vi "LVObject to JSON.vi"(5 "enable LabVIEW extensions? (T)":bool=TRUE, 6 "Pretty Print?":bool, 7 "JSON Serializable Serializer in":refnum<class "JSON Serializable Serializer.lvclass">, 8 "error in (no error)":errorcluster, 10 "Object":refnum<class>) -> (0 "error out":errorcluster, 2 "<JSON>Object":string)   [LabVIEW 2017, in "JSON Serializable Serializer.lvclass"]
uses:
  JSON Serializable Serializer.lvclass
  C:/Program Files (x86)/National Instruments/LabVIEW 2017/vi.lib/JDP Science/JSONtext/LVClass Serializer/JSONtext LVClass Serializer.lvclass
  JSON Serializable/JSON Serializable.lvclass
  Default Serialization Binder/Default Serialization Binder.lvclass
  <vilib>/JDP Science/JSONtext/Set Multiple Object Items.vi
  <vilib>/JDP Science/JSONtext/Get all Object Items.vi
  <vilib>/JDP Science/JSONtext/JSON type.vi
  <vilib>/JDP Science/JSONtext/JSONtext.lvlib
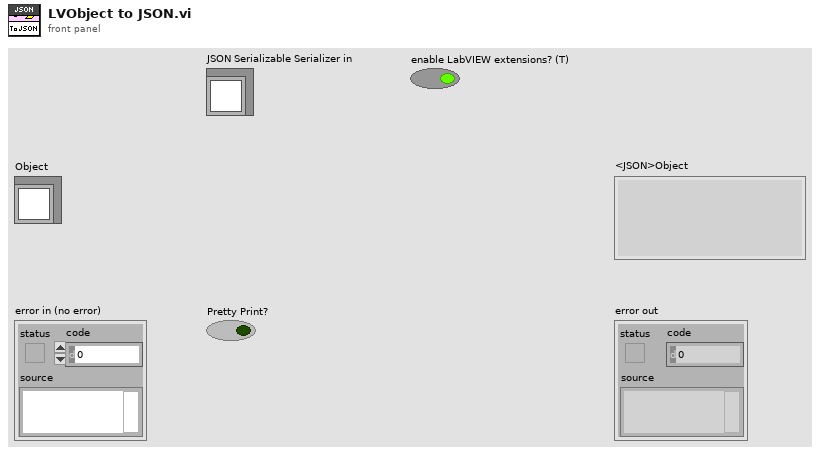
[diagram p1: front panel]
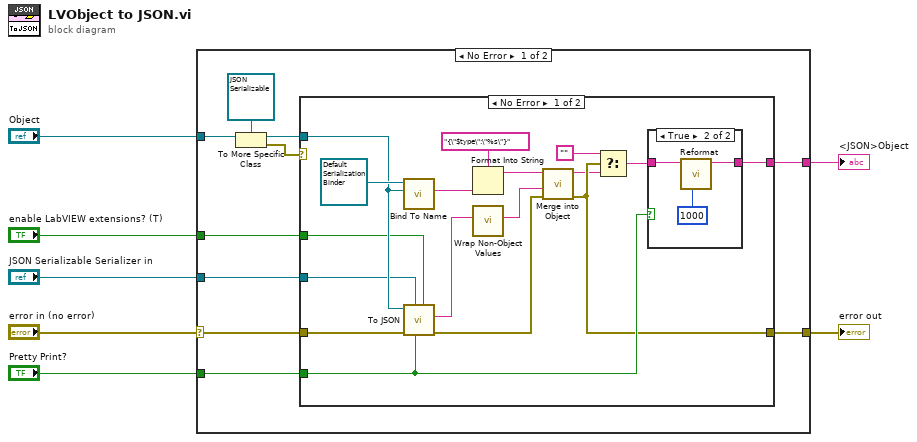
[diagram p0: block diagram]
diagram:
  n1 = case shown="No Error" "error in (no error)" {
    selector: "error in (no error)" -> [w9 w40]
    tunnel: [w17 _] -> w7
    tunnel: "Object" -> [w16 _]
    tunnel: [w8 w40] -> w5
    tunnel: "Pretty Print?" -> [w12 _]
    tunnel: "JSON Serializable Serializer in" -> [w11 _]
    tunnel: "enable LabVIEW extensions? (T)" -> [w10 _]
    frame No Error {
      n2 = To More Specific Class(target class=refnum<class "JSON Serializable.lvclass"> refnum ("JSON Serializable.lvclass"), reference=w16) -> (specific class reference=w14:refnum<class "JSON Serializable.lvclass">, error out=w13:errorcluster)  [unwired: 1 in]
      n3 = case shown="No Error" w13 {
        tunnel: [w18 _] -> w17
        tunnel: w14 -> [w31 _]
        tunnel: w12 -> [w25 _]
        tunnel: w11 -> [w26 _]
        tunnel: w10 -> [w29 _]
        tunnel: w9 -> [w28 w39]
        tunnel: [w22 w39] -> w8
        frame No Error {
          n4 = call-dynamic "Bind To Name.vi"("Type"=w31, "Default Serialization Binder in"=refnum<class "Default Serialization Binder.lvclass"> refnum ("Default Serialization Binder")) -> ("Type Name"=w33:string)  [unwired: 7 in, 2 out]
          n5 = call-dynamic "To JSON.vi"("enable LabVIEW extensions? (T)"=w29, "Pretty Print?"=w25, "LVClass Serializer"=w26, "error in (no error)"=w28, "JSON Serializable in"=w31) -> ("error out"=w27:errorcluster, "<JSON>"=w23:string)  [unwired: 4 in, 1 out]
          n6 = Format Into String(format string="{\"$type\":\"%s\"}", w33) -> (resulting string=w30:string)  [unwired: 2 in, 1 out]
          n7 = call "Wrap Non-Object Values.vi"("<JSON> in"=w23) -> ("<JSON> out"=w24:string)  [unwired: 10 in]
          n8 = call <vilib>:"Merge into Object.vi"("error in (no error)"=w27, "JSON Object to Merge"=w24, "JSON"=w30) -> ("error out"=w22:errorcluster, "<JSON>"=w20:string)  [unwired: 6 in]
          n9 = Select(t="", s=w22, f=w20) -> (s? t:f=w19:string)
          n10 = case shown="True" w25 {
            tunnel: w19 -> [w35 w38]
            tunnel: [w35 w37] -> w18
            frame False {
            }
            frame True {
              n11 = call <vilib>:"Reformat.vi"("Pretty Print Levels"=1000, "JSON"=w38) -> ("<JSON>"=w37:string)  [unwired: 6 in, 3 out]
            }
          }
        }
        frame Error {
        }
      }
    }
    frame Error {
    }
  }
  "error out" <- w5
  "<JSON>Object" <- w7
